vi "Get Center Frequency.vi"(8 "error in (no error)":errorcluster, 11 "DeviceRefnum":u64) -> (0 "error out":errorcluster, 2 "Center Frequency":dbl, 3 "DeviceRefnum Out":u64)   [LabVIEW 2014]
doc: "Gets actual frequency the device is tuned to in Hz."
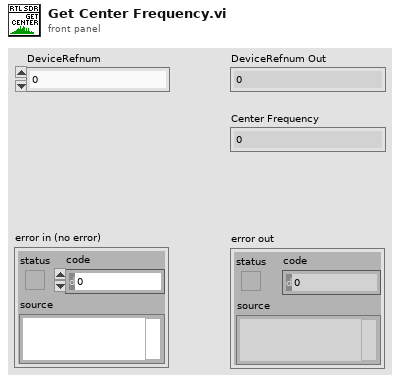
[diagram p1: front panel]
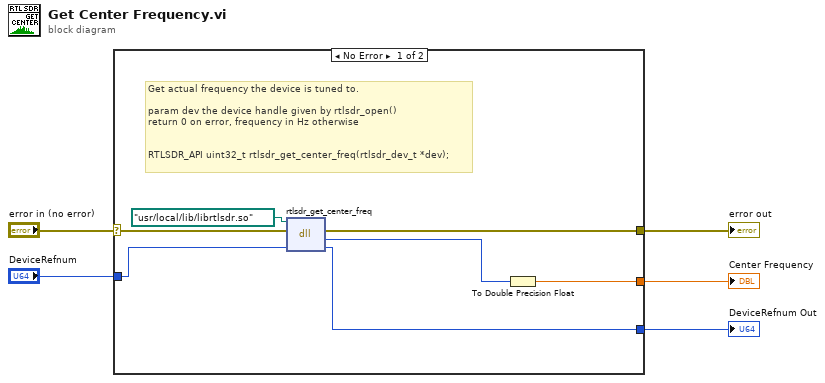
[diagram p0: block diagram]
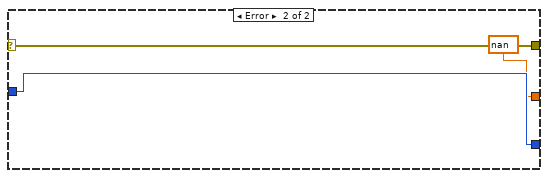
[diagram p2: hidden frame]
diagram:
  n1 = case shown="No Error" "error in (no error)" {
    selector: "error in (no error)" -> [w9 w15]
    tunnel: [w7 w15] -> w5
    tunnel: "DeviceRefnum" -> [w12 w14]
    tunnel: [w11 w14] -> w3
    tunnel: [w6 nan] -> w2
    frame No Error {
      # "Get actual frequency the device is tuned to.\n\nparam dev the device handle given by rtlsdr_open()\nreturn 0 on error, frequency in Hz otherwise\n\n\nRTLSDR_API uint32_t rtlsdr_get_center_freq(rtlsdr_dev_t *dev);"
      n2 = dll-call lib="C:/Program Files (x86)/National Instruments/LabVIEW 2016/user.lib/rtlsdr/rtlsdr.*" fn="rtlsdr_get_center_freq"(path in=path "/usr/local/lib/librtlsdr.so", error in=w9, "DeviceRefnum"=w12) -> (error out=w7:errorcluster, "return type"=w10:u32, "DeviceRefnum"=w11:u64)  [unwired: 1 in, 1 out]
      n3 = To Double Precision Float(number=w10) -> (double precision float=w6:dbl)
    }
    frame Error {
    }
  }
  "error out" <- w5
  "DeviceRefnum Out" <- w3
  "Center Frequency" <- w2
